vi "Wait UI.vi"(8 "error in (no error)":errorcluster, 9 "Timeout mSec (-1)":i32=-1, 11 "Bar in":refnum<class "Bar.lvclass">) -> (0 "error out":errorcluster, 1 "Timed Out ?":bool, 2 "No Wait ?":bool, 3 "Bar out":refnum<class "Bar.lvclass">)   [LabVIEW 2015, in "Simple Progress Bar.lvlib" / "Bar.lvclass"]
uses:
  Bar.lvclass
  Bar.lvclass/Bar.ctl
panel:
  out "Waiting for User":bool
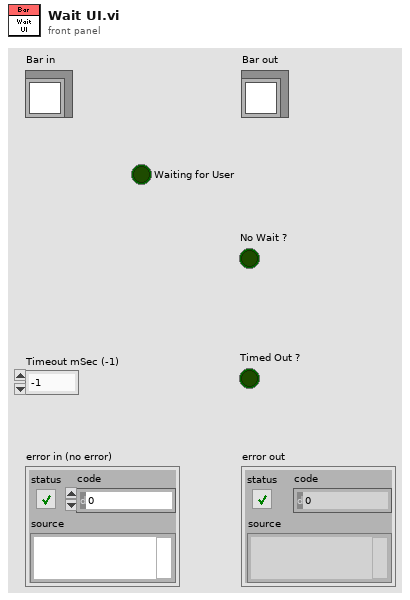
[diagram p1: front panel]
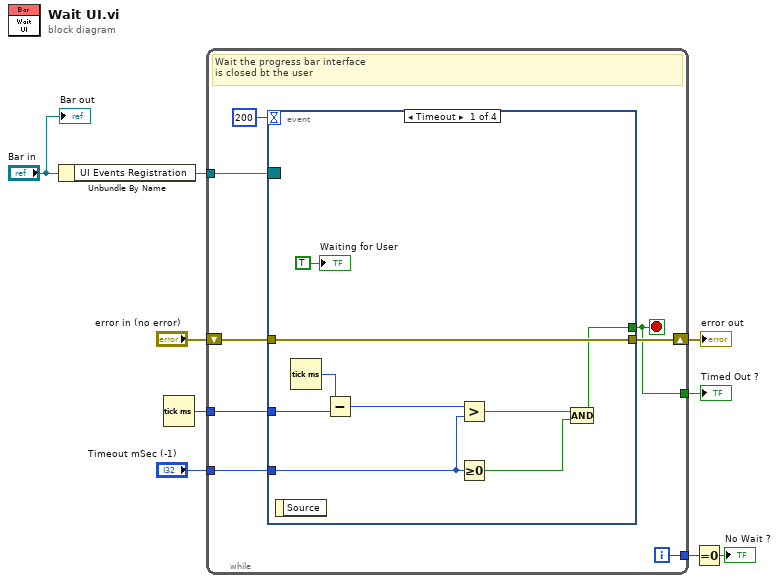
[diagram p0: block diagram]
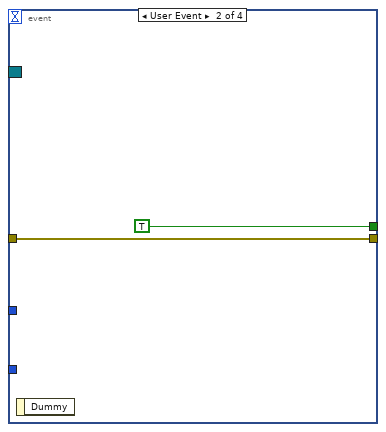
[diagram p2: hidden frame]
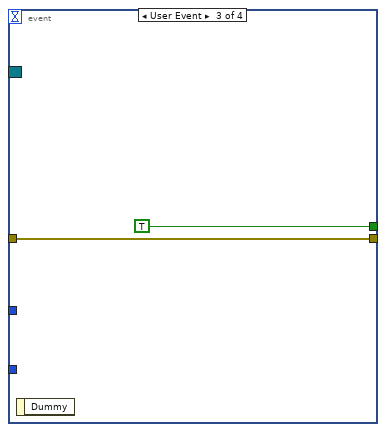
[diagram p3: hidden frame]
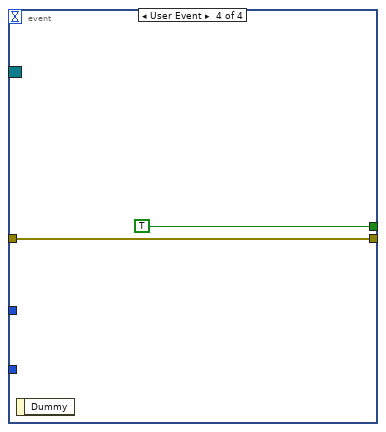
[diagram p4: hidden frame]
diagram:
  n1 = Unbundle By Name("Bar in") -> ("UI Events Registration"=w2:refnum<event-registration>)
  n2 = Tick Count (ms)() -> (millisecond timer value=w7:u32)
  n3 = while {
    shift-right: [w16] -> w8
    shift-left: "error in (no error)" -> [w17]
    tunnel: w2 -> [w14]
    tunnel: w7 -> [w13]
    tunnel: "Timeout mSec (-1)" -> [w12]
    tunnel: [w11] -> w5
    tunnel: [w10] -> w4
    i -> [w10]
    stop <- w11 stop-if-true
    # "Wait the progress bar interface\nis closed bt the user"
    n4 = event shown="[0] Timeout" {
      selector: w14 -> [_ _ _ _]
      dyn-events: _ -> [_ _ _ _]
      timeout: 200 -> [_ _ _ _]
      tunnel: [w26 w28 w29 w31] -> w16
      tunnel: w17 -> [w26 w28 w29 w31]
      tunnel: [w20 TRUE TRUE TRUE] -> w11
      tunnel: w13 -> [w23 _ _ _]
      tunnel: w12 -> [w19 _ _ _]
      event Timeout {
        n5 = event-data() -> ()  [unwired: 1 in, 1 out]
        n6 = Tick Count (ms)() -> (millisecond timer value=w24:u32)
        n7 = Subtract(x=w24, y=w23) -> (x-y=w22:u32)
        n8 = Greater?(x=w22, y=w19) -> (0:w21:bool)
        n9 = Greater Or Equal To 0?(x=w19) -> (x >= 0?=w18:bool)
        n10 = Compound Arithmetic op=AND(w21, w18) -> (w20:bool)
        "Waiting for User" <- TRUE ("Waiting for User")
      }
      event User Event {
        n11 = event-data() -> ()  [unwired: 1 in, 1 out]
      }
      event User Event {
        n12 = event-data() -> ()  [unwired: 1 in, 1 out]
      }
      event User Event {
        n13 = event-data() -> ()  [unwired: 1 in, 1 out]
      }
    }
  }
  "error out" <- w8
  "Timed Out ?" <- w5
  n14 = Equal To 0?(x=w4) -> (x = 0?=→"No Wait ?":bool)
  "Bar out" <- "Bar in"
